vi "Xml_Load_Default.vi"(8 "error in (no error)":errorcluster, 11 "Variant":variant) -> (0 "error out":errorcluster)   [LabVIEW 2024]
doc: "This VI reads a XML parameter file and fills the controls and indicators of the UI panel. \nA full experiment can start immediattely after loading the XML file.\n\n1. Open a XML file. By default propose to open the last.xml file, but the user can choose any other file.\n2. Read the version of XML schema. \n3. The controls of the main UI panel are passed by reference through the QMH UI Cluster and updated with the values read into the XML file."
uses:
  controls/QMH_UI_Cluster.ctl
  controls/QMH_UI_References.ctl
  controls/QMH_UI_Report.ctl
  controls/QMH_UI_Command.ctl
  controls/QMH_ICR_Command.ctl
  controls/QMH_Status.ctl
  controls/EXPERT_Path_Selector.ctl
  Global_Variables.vi
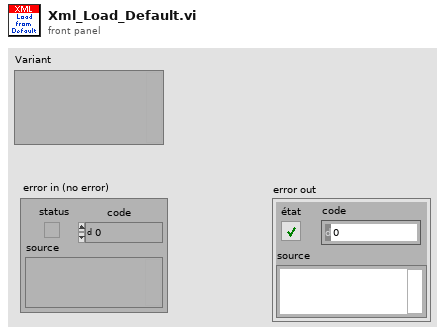
[diagram p1: front panel]
types:
  T1 = typedef "EXPERT_Path_Selector.ctl" = enum16{"Application", "Resources", "Data", "XML", "XML Saved", "Load Directory"}
  T2 = typedef "QMH_UI_Cluster.ctl" = cluster{"QMH UI References":T3, "QMH UI Report":T4}
  T3 = typedef "QMH_UI_References.ctl" = cluster{"Refnum Load":refnum<vi>, "Refnum Save As":refnum<vi>, "Refnum Start":refnum<vi>, "Refnum Exit":refnum<vi>, "Refnum Tabs":refnum<vi>, "Refnum SPECTRUM":refnum<vi>, "Refnum EXPERIMENT":refnum<vi>, "Refnum VOLTAGES":refnum<vi>, "Refnum SEQUENCE":refnum<vi>, "Refnum EXPERT":refnum<vi>, "Refnum LOOPS":refnum<vi>, "Refnum EXCIT Table":refnum<vi>, "Refnum TIMING Table":refnum<vi>, "Refnum CHANGE Experiment":refnum<vi>, "Refnum CHANGE Voltages":refnum<vi>, "Refnum CHANGE Sequence":refnum<vi>, "Refnum CHANGE Expert":refnum<vi>, "Refnum CHANGE Loops":refnum<vi>, "Refnum CHANGE Scientist":refnum<vi>, "Refnum PIL Status":refnum<vi>}
  T4 = typedef "QMH_UI_Report.ctl" = cluster{"UI Status":T5, "ICR Status":T6, "QMH Status":T7}
  T5 = typedef "QMH_UI_Command.ctl" = enum16{"Initialize", "UI Load", "UI Save", "UI Save As", "UI Change Experiment", "UI Change Voltages", "UI Change Sequence", "UI Change Expert", "UI Change Loops", "UI Change Scientist", "Ready to Start", "UI Start", "Waiting for ICR", "UI Exit", "Update Experiment", "Update Report", "Update ICR Status", "Waiting for User"}
  T6 = typedef "QMH_ICR_Command.ctl" = enum16{"Initialize", "Sequence Loop Setup", "Sequence Setup", "ICR Start", "ICR Stop", "Hardware Setup", "Next Sequence Loop", "Next Accumulation", "Waiting for Trigger", "Sequence Started", "Sequence Finished", "Sequence Loop Done", "Writing Data", "Hardware Reset", "Exit"}
  T7 = typedef "QMH_Status.ctl" = enum16{"Init", "Loading", "Setup", "Ready to Start", "Started", "Idle"}
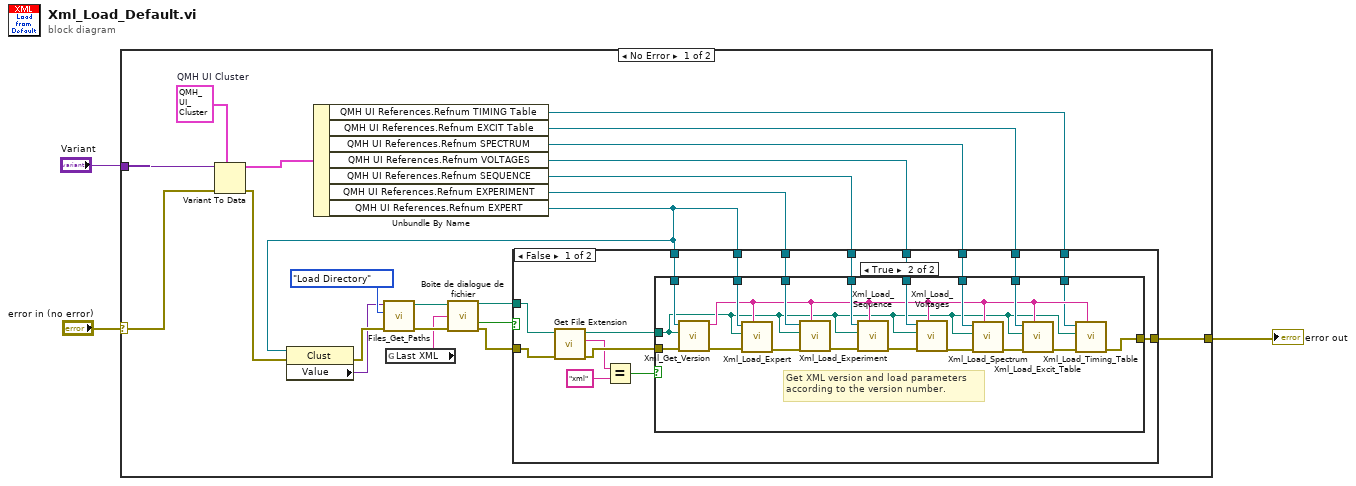
[diagram p0: block diagram]
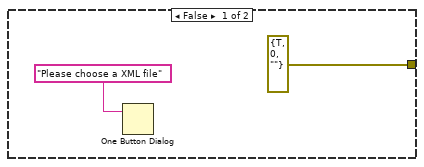
[diagram p2: hidden frame]
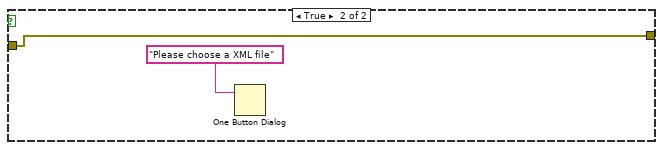
[diagram p3: hidden frame]
diagram:
  n1 = case shown="No Error" "error in (no error)" {
    selector: "error in (no error)" -> [w24 w65]
    tunnel: "Variant" -> [w17 _]
    tunnel: [w19 w65] -> w2
    frame No Error {
      w25 = T2 {"QMH UI References"={"Refnum Load"=refnum, "Refnum Save As"=refnum, "Refnum Start"=refnum, "Refnum Exit"=refnum, "Refnum Tabs"=refnum, "Refnum SPECTRUM"=refnum, "Refnum EXPERIMENT"=refnum, "Refnum VOLTAGES"=refnum, "Refnum SEQUENCE"=refnum, "Refnum EXPERT"=refnum, "Refnum LOOPS"=refnum, "Refnum EXCIT Table"=refnum, "Refnum TIMING Table"=refnum, "Refnum CHANGE Experiment"=refnum, "Refnum CHANGE Voltages"=refnum, "Refnum CHANGE Sequence"=refnum, "Refnum CHANGE Expert"=refnum, "Refnum CHANGE Loops"=refnum, "Refnum CHANGE Scientist"=refnum, "Refnum PIL Status"=refnum}, "QMH UI Report"={"UI Status"=enum."Initialize", "ICR Status"=enum."Initialize", "QMH Status"=enum."Init"}}  # QMH UI Cluster
      n2 = Variant To Data(error in=w24, type=w25, Variant=w17) -> (data=w20:T2, error out=w14:errorcluster)
      n3 = Unbundle By Name(w20) -> ("QMH UI References.Refnum TIMING Table"=w5:refnum<vi>, "QMH UI References.Refnum EXCIT Table"=w6:refnum<vi>, "QMH UI References.Refnum SPECTRUM"=w7:refnum<vi>, "QMH UI References.Refnum VOLTAGES"=w23:refnum<vi>, "QMH UI References.Refnum SEQUENCE"=w22:refnum<vi>, "QMH UI References.Refnum EXPERIMENT"=w21:refnum<vi>, "QMH UI References.Refnum EXPERT"=w4:refnum<vi>)
      n4 = property class="Clust"(reference=w4, error in=w14) -> (error out=w13:errorcluster, "Value"=w8:variant)  [unwired: 1 out]
      n5 = call "Files_Get_Paths.vi"("error in (no error)"=w13, "EXPERT Path Selector"=EXPERT_Path_Selector."Load Directory", "Variant"=w8) -> ("error out"=w18:errorcluster, "Path"=w16:path)  [unwired: 7 in]
      n6 = global read "Global_Variables.vi" "Last XML"() -> (w12:string)
      n7 = call "Boîte de dialogue de fichier"("start path"=w16, "default name"=w12, "error in"=w18) -> ("selected path"=w11:path, "cancelled"=w9:bool, "error out"=w10:errorcluster)  [unwired: 9 in, 1 out]
      n8 = case shown="False" w9 {
        tunnel: w23 -> [w41 _]
        tunnel: w22 -> [w40 _]
        tunnel: w21 -> [w39 _]
        tunnel: w4 -> [w38 _]
        tunnel: [w37 w63] -> w19
        tunnel: w7 -> [w36 _]
        tunnel: w4 -> [w35 _]
        tunnel: w11 -> [w34 _]
        tunnel: w10 -> [w32 w63]
        tunnel: w6 -> [w27 _]
        tunnel: w5 -> [w26 _]
        frame False {
          n9 = call <vilib>:"Get File Extension.vi"("error in (no error)"=w32, "file"=w34) -> ("error out"=w31:errorcluster, "lowercase file extension"=w30:string, "dup file"=w33:path)  [unwired: 5 in, 2 out]
          n10 = Equal?(x=w30, y="xml") -> (x = y?=w28:bool)
          n11 = case shown="True" w28 {
            tunnel: w41 -> [_ w62]
            tunnel: w40 -> [_ w61]
            tunnel: w39 -> [_ w60]
            tunnel: w38 -> [_ w59]
            tunnel: [errorcluster {"status"=TRUE, "code"=0, "source"=""} ("error out") w47] -> w37
            tunnel: w36 -> [_ w52]
            tunnel: w35 -> [_ w51]
            tunnel: w33 -> [_ w44]
            tunnel: w31 -> [_ w50]
            tunnel: w27 -> [_ w48]
            tunnel: w26 -> [_ w45]
            frame False {
              n12 = One Button Dialog(message="Please choose a XML file") -> ()  [unwired: 1 in, 1 out]
            }
            frame True {
              # "Get XML version and load parameters\naccording to the version number."
              n13 = call "Xml_Get_Version.vi"("error in (no error)"=w50, "XML Path"=w44, "Refnum Cluster"=w51) -> ("error out"=w54:errorcluster, "Version String"=w46:string)  [unwired: 7 in]
              n14 = call "Xml_Load_Expert.vi"("Version String"=w46, "error in (no error)"=w54, "XML Path"=w44, "Refnum Clust"=w59) -> ("error out"=w53:errorcluster)  [unwired: 7 in]
              n15 = call "Xml_Load_Experiment.vi"("Version String"=w46, "error in (no error)"=w53, "XML Path"=w44, "Refnum Clust"=w60) -> ("error out"=w57:errorcluster)  [unwired: 7 in]
              n16 = call "Xml_Load_Sequence.vi"("Version String"=w46, "error in (no error)"=w57, "XML Path"=w44, "Refnum Clust"=w61) -> ("error out"=w56:errorcluster)  [unwired: 7 in]
              n17 = call "Xml_Load_Voltages.vi"("Version String"=w46, "error in (no error)"=w56, "XML Path"=w44, "Refnum Clust"=w62) -> ("error out"=w55:errorcluster)  [unwired: 7 in]
              n18 = call "Xml_Load_Spectrum.vi"("Version String"=w46, "error in (no error)"=w55, "XML Path"=w44, "Refnum Clust"=w52) -> ("error out"=w58:errorcluster)  [unwired: 7 in]
              n19 = call "Xml_Load_Excit_Table.vi"("Version String"=w46, "error in (no error)"=w58, "XML Path"=w44, "Refnum Clust"=w48) -> ("error out"=w49:errorcluster)  [unwired: 7 in]
              n20 = call "Xml_Load_Timing_Table.vi"("Version String"=w46, "error in (no error)"=w49, "XML Path"=w44, "Refnum Clust"=w45) -> ("error out"=w47:errorcluster)  [unwired: 7 in]
            }
          }
        }
        frame True {
          n21 = One Button Dialog(message="Please choose a XML file") -> ()  [unwired: 1 in, 1 out]
        }
      }
    }
    frame Error {
    }
  }
  "error out" <- w2
